vi "Write.vi"(8 "error in (no error)":errorcluster, 10 "Data":string, 11 "Mock Instrument Interface in":refnum<class "Mock Instrument.lvclass">) -> (0 "error out":errorcluster, 3 "Mock Instrument Interface out":refnum<class "Mock Instrument.lvclass">)   [LabVIEW 2020, in "Low Level PSU With Tests.lvlib" / "Mock Instrument.lvclass"]
uses:
  Mock Instrument.lvclass
  Mock Instrument.lvclass/Mock Instrument.ctl
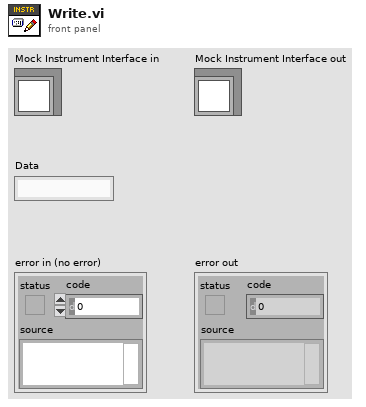
[diagram p1: front panel]
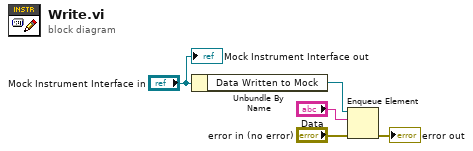
[diagram p0: block diagram]
diagram:
  n1 = Unbundle By Name("Mock Instrument Interface in") -> ("Data Written to Mock"=w4:refnum<queue>)
  n2 = Enqueue Element(queue=w4, element="Data", error in (no error)="error in (no error)") -> (error out=→"error out":errorcluster)  [unwired: 1 in, 2 out]
  "Mock Instrument Interface out" <- "Mock Instrument Interface in"
